vi "Main Listen for TCP Commands.vi"(8 "error in (no error)":errorcluster, 11 "J1939 Main Configuration":T1={"Parameters"={"J1939 XNET Settings"={"XNET Database"="", "XNET Cluster"="", "CAN Port"="", "Baud rate [Bd]"=0, "Termination"=0, "Incoming Rate"=0, "Outcoming Rate"=1, "Write Decimation"=1}, "Incoming Single Point Configuraiton"={"Incoming Single Point Frame"={"ID"=[], "Conversion"=[], "Channel Array Positions"=[], "Frame Length"=[]}, "Channel Pairs"={"Chan Refs"=[], "Previous Chan Values"=[]}, "Read FIFO"=refnum}, "Outgoing Cyclic Configuraiton"={"Outgoing Cyclic Frame"={"ID"=[], "Conversion"=[], "Channel Array Positions"=[], "Frame Length"=[], "Transmit Propreties"=[]}, "Channel Pairs"={"Block Data Refs"=[], "Previous Chan Values"=[]}, "Write FIFO"=refnum}, "J1939 Monitor Settings"={"J1939 Network Address"=0, "Name"=0}, "Simulated Addresses"=[], "Simulated Addresses LUT"=variant, "Name"=""}, "Name"="", "J1939 Cluster"={"Processed Incoming"=refnum, "Current Device Address"=0, "Processed Outgoing"=refnum, "Process Outgoing"=refnum, "Name"=0}, "References"={"BAM Buffer"=refnum, "CM Buffer"=refnum, "CM Gen"=refnum, "BAM Gen"=refnum, "Address Claims"=refnum, "RQST"=refnum}, "Frame In"="", "Frame Out"="", "Incoming Timeout"=0, "Outgoing Timeout"=0, "Listener ID"=refnum, "Process"=refnum, "Data Ref"=refnum, "Scale Ref"=refnum, "Incoming Direct Access"={"Offset"=0, "Length"=0}, "Outgoing Direct Access"={"Offset"=0, "Length"=0}, "TCP Mngr Ref"=refnum, "Name and Address"="", "Simulated Addresses"=[], "Simulated Addresses LUT"=variant} {"Simulated Addresses"."Simulated Addresses"."J1939 XNET Settings"."Name" format="%.0x"; "Simulated Addresses"."Simulated Addresses"."DM1 Data"."Data Reference" format="%.0x"; "Simulated Addresses"."Simulated Addresses"."DM1 Enable?"."Data Reference" format="%.0x"; "Simulated Addresses"."Simulated Addresses"."DM2 Data"."Data Reference" format="%.0x"; "Simulated Addresses"."Simulated Addresses"."DM2 Enable?"."Data Reference" format="%.0x"; "Parameters"."Simulated Addresses"."Simulated Addresses"."J1939 XNET Settings"."Name" format="%.0x"; "Parameters"."J1939 Monitor Settings"."Name" format="%.0x"; "Parameters"."Outgoing Cyclic Configuraiton"."Channel Pairs"."Block Data Refs"."Data Reference" format="%.0x"; "Parameters"."Outgoing Cyclic Configuraiton"."Outgoing Cyclic Frame"."Transmit Propreties"."Transmit Time" format="%#_p"; "Parameters"."J1939 XNET Settings"."Termination" items=["Off", "On"]; "Parameters"."Incoming Single Point Configuraiton"."Channel Pairs"."Chan Refs" format="%.0x"}) -> (0 "error out":errorcluster)   [LabVIEW 2015, in "J1939 Addon Engine.lvlib"]
uses:
  J1939 Addon Engine.lvlib
  Types/Configuration Cluster.ctl
  <vilib>/NI/NI VeriStand Inline Async API/_VS Inline Async API/Process/Process.lvclass
  Types/Process Parameters.ctl
  Shared/Types/XNET Settings.ctl
  Types/Incoming Single Point Configuration.ctl
  Types/Incoming Single Point Frame Pairs.ctl
  Shared/Types/Incoming Single Point Channel Pairs.ctl
  <vilib>/NI Veristand/Custom Device API/Data Reference.ctl
  Types/Outgoing Cyclic Configuration.ctl
  Types/Outgoing Cyclic Frame Pairs.ctl
  Shared/Types/XNET Frame Event Properties.ctl
  Shared/Types/Outgoing Cyclic Channel Pairs.ctl
  <vilib>/NI Veristand/Custom Device API/Block Data Reference.ctl
  Shared/Types/Monitor Settings.ctl
  Types/Simulated Settings.ctl
  Shared/Types/Compiled Simulated Settings.ctl
  Types/DTC FIFOs.ctl
  J1939 Multi Packet Frame/Types/Setup Information Cluster.ctl
  <vilib>/xnet/xnet.llb/XNET Frame CAN.ctl
  <vilib>/xnet/xnet.llb/XNET Frame Type CAN.ctl
  Shared/J1939 Utilities/Types/CAN Outgoing Message Cluster.ctl
  J1939 Multi Packet Frame/Types/TP List References.ctl
  J1939 Multi Packet Frame/Types/BAM Buffer Connections List_Ref.ctl
  J1939 Multi Packet Frame/Types/TP Buffer Connection Cluster.ctl
  J1939 Multi Packet Frame/Types/Connection Mode Generation Connection Ref.ctl
  J1939 Multi Packet Frame/Types/Connection Mode Generation Connection Cluster.ctl
  J1939 Multi Packet Frame/Types/BAM Generation Connections List_Ref.ctl
  J1939 Multi Packet Frame/Types/BAM Generation Connection Cluster.ctl
  J1939 Multi Packet Frame/Types/Address Table Reference.ctl
  J1939 Multi Packet Frame/Types/RQST Lookup Table Reference.ctl
  Types/Data Lookup Table Reference.ctl
  Types/Datatable Lookup DVR.ctl
  Types/Conversion Lookup Table Reference.ctl
  Shared/Types/RQST Comm Lookup Table_Ref.ctl
  Shared/STM/Connection Manager/stm_ManagerStateVariables.ctl
  Shared/STM/TCP/stm_TCP Connection Info.ctl
  Shared/STM/_SubVIs/stm_MetaDataElement.ctl
  Shared/STM/Connection Manager/stm_TCPConnectionProperties.ctl
  Shared/STM/Connection Manager/stm_TCPConnectionMethod.ctl
  Shared/STM/TCP/stm_TCP Read Options.ctl
  Shared/Types/Request Message.ctl
  J1939 Multi Packet Frame/Types/Address Lookup Table Action.ctl
  <vilib>/NI/NI VeriStand Inline Async API/_VS Inline Async API/Process/Process.lvclass/Process.ctl
  Shared/STM/TCP/STM Get Connection Reference (TCP).vi
  Shared/J1939 Utilities/Common Messages.vi
  Shared/J1939 Utilities/SubVIs/Request.vi
  J1939 Multi Packet Frame/SubVIs/RQST Lookup Table Act.vi
  <vilib>/NI/NI VeriStand Inline Async API/_VS Inline Async API/Error Handling Process/SubVIs/Error.ConvertArray.vi
  Shared/J1939 Utilities/Common Conversions.vi
  Shared/J1939 Utilities/SubVIs/Convert J1939 ID to CAN Arb ID.vi
  Shared/STM/Connection Manager/TCP Connection Manager.vi
  Shared/STM/TCP/STM Write Message (TCP).vi
  J1939 Multi Packet Frame/SubVIs/Address Lookup Table.vi
  <vilib>/xnet/xnet.llb/XNET Read (State CAN Comm).vi
  J1939 Multi Packet Frame/SubVIs/RQST Lookup Table.vi
  Shared/STM/TCP/STM Read Message (TCP).vi
  Shared/J1939 Addon Shared.lvlib
  Shared/J1939 Utilities/J1939 Utilities.lvlib
  <vilib>/NI Veristand/Custom Device Tools/Custom Device Utility Library/Custom Device Utility Library.lvlib
  <vilib>/NI VeriStand/Custom Device API/Custom Device API.lvlib
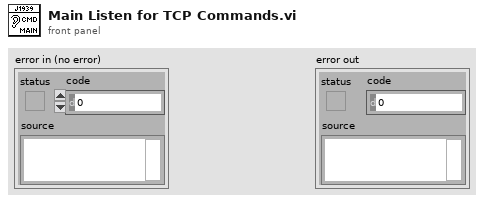
[diagram p1: front panel]
types:
  T1 = typedef "J1939 Addon Engine.lvlib/Configuration Cluster.ctl" = cluster{"Parameters":T2, "Name":string, "J1939 Cluster":T17, "References":T18, "Frame In":refnum<k21>, "Frame Out":refnum<k21>, "Incoming Timeout":u32, "Outgoing Timeout":u32, "Listener ID":refnum<k5>, "Process":refnum<class "Process.lvclass">, "Data Ref":T24, "Scale Ref":T25, "Incoming Direct Access":cluster{"Offset":u32, "Length":u32}, "Outgoing Direct Access":cluster{"Offset":u32, "Length":u32}, "TCP Mngr Ref":T26, "Name and Address":string, "Simulated Addresses":T14[], "Simulated Addresses LUT":variant}
  T2 = typedef "J1939 Addon Engine.lvlib/Process Parameters.ctl" = cluster{"J1939 XNET Settings":T3, "Incoming Single Point Configuraiton":T4, "Outgoing Cyclic Configuraiton":T8, "J1939 Monitor Settings":T13, "Simulated Addresses":T14[], "Simulated Addresses LUT":variant, "Name":string}
  T3 = typedef "J1939 Addon Shared.lvlib/XNET Settings.ctl" = cluster{"XNET Database":refnum<k21>, "XNET Cluster":refnum<k21>, "CAN Port":string, "Baud rate [Bd]":u32, "Termination":u32, "Incoming Rate":u32, "Outcoming Rate":u32, "Write Decimation":u32}
  T4 = typedef "J1939 Addon Engine.lvlib/Incoming Single Point Configuration.ctl" = cluster{"Incoming Single Point Frame":T5, "Channel Pairs":T6, "Read FIFO":refnum<k33>}
  T5 = typedef "J1939 Addon Engine.lvlib/Incoming Single Point Frame Pairs.ctl" = cluster{"ID":u32[], "Conversion":refnum<k21>[], "Channel Array Positions":cluster{"Offset":u32, "Length":u32}[], "Frame Length":u32[]}
  T6 = typedef "J1939 Addon Shared.lvlib/Incoming Single Point Channel Pairs.ctl" = cluster{"Chan Refs":T7[], "Previous Chan Values":dbl[]}
  T7 = typedef "Custom Device API.lvlib/Data Reference.ctl" = i32
  T8 = typedef "J1939 Addon Engine.lvlib/Outgoing Cyclic Configuration.ctl" = cluster{"Outgoing Cyclic Frame":T9, "Channel Pairs":T11, "Write FIFO":refnum<k33>}
  T9 = typedef "J1939 Addon Engine.lvlib/Outgoing Cyclic Frame Pairs.ctl" = cluster{"ID":u32[], "Conversion":refnum<k21>[], "Channel Array Positions":cluster{"Offset":u32, "Length":u32}[], "Frame Length":u32[], "Transmit Propreties":T10[]}
  T10 = typedef "J1939 Addon Shared.lvlib/XNET Frame Event Properties.ctl" = cluster{"Transmit trigger":enum16{"Channel value change"}, "Enable software cyclic trigger":bool, "Transmit Time":dbl}
  T11 = typedef "J1939 Addon Shared.lvlib/Outgoing Cyclic Channel Pairs.ctl" = cluster{"Block Data Refs":T12[], "Previous Chan Values":dbl[]}
  T12 = typedef "Custom Device API.lvlib/Block Data Reference.ctl" = cluster{"Data Reference":T7, "Offset":u64, "Length":u64}
  T13 = typedef "J1939 Addon Shared.lvlib/Monitor Settings.ctl" = cluster{"J1939 Network Address":u8, "Name":u64}
  T14 = typedef "J1939 Addon Engine.lvlib/Simulated Settings.ctl" = cluster{"Simulated Addresses":T15, "FIFOs":T16}
  T15 = typedef "J1939 Addon Shared.lvlib/Compiled Simulated Settings.ctl" = cluster{"J1939 XNET Settings":T13, "DM1 Data":T12[], "DM1 Data":dbl[], "DM1 Enable?":T12[], "DM1 Enable?":dbl[], "DM2 Data":T12[], "DM2 Data":dbl[], "DM2 Enable?":T12[], "DM2 Enable?":dbl[]}
  T16 = typedef "J1939 Addon Engine.lvlib/DTC FIFOs.ctl" = cluster{"DM1 Data":refnum<k33>, "DM1 Enable?":refnum<k33>, "DM2 Data":refnum<k33>, "DM2 Enable?":refnum<k33>, "DM1 Reset?":refnum<k33>, "DM2 Reset?":refnum<k33>}
  T17 = typedef "J1939 Addon Engine.lvlib/Setup Information Cluster.ctl" = cluster{"Processed Incoming":refnum<queue>, "Current Device Address":u8, "Processed Outgoing":refnum<queue>, "Process Outgoing":refnum<queue>, "Name":u64}
  T18 = typedef "J1939 Addon Engine.lvlib/TP List References.ctl" = cluster{"BAM Buffer":T19, "CM Buffer":T19, "CM Gen":T20, "BAM Gen":T21, "Address Claims":T22, "RQST":T23}
  T19 = typedef "J1939 Addon Engine.lvlib/BAM Buffer Connections List_Ref.ctl" = refnum<data-value>
  T20 = typedef "J1939 Addon Engine.lvlib/Connection Mode Generation Connection Ref.ctl" = refnum<data-value>
  T21 = typedef "J1939 Addon Engine.lvlib/BAM Generation Connections List_Ref.ctl" = refnum<data-value>
  T22 = typedef "J1939 Addon Engine.lvlib/Address Table Reference.ctl" = refnum<data-value>
  T23 = typedef "J1939 Addon Engine.lvlib/RQST Lookup Table Reference.ctl" = refnum<data-value>
  T24 = typedef "J1939 Addon Engine.lvlib/Data Lookup Table Reference.ctl" = refnum<data-value>
  T25 = typedef "J1939 Addon Engine.lvlib/Conversion Lookup Table Reference.ctl" = refnum<data-value>
  T26 = typedef "J1939 Addon Shared.lvlib/RQST Comm Lookup Table_Ref.ctl" = refnum<data-value>
  T27 = typedef "J1939 Addon Shared.lvlib/stm_TCPConnectionMethod.ctl" = enum16{"Initialize", "Add Connection", "Set Properties", "Get Connection(s)", "Remove Connection", "Remove All Connections", "Get Connection Count"}
  T28 = typedef "J1939 Addon Shared.lvlib/stm_TCP Read Options.ctl" = cluster{"Ignore Timeout Error":bool, "timeout ms (1000)":i32}
  T29 = typedef "J1939 Addon Shared.lvlib/Request Message.ctl" = cluster{"PGN":u32, "DA":u8, "Ignore Response":bool}
  T30 = typedef "J1939 Addon Shared.lvlib/J1939 Utilities.lvlib/CAN Outgoing Message Cluster.ctl" = cluster{"Identifier":u32, "Data":u8[]}
  T31 = typedef "J1939 Addon Engine.lvlib/Address Lookup Table Action.ctl" = enum16{"Initialize", "Add", "Get", "Remove", "Get All"}
  T32 = typedef "J1939 Addon Shared.lvlib/stm_TCP Connection Info.ctl" = cluster{"connection ID":refnum<k5>, "Meta data":T33[]}
  T33 = typedef "J1939 Addon Shared.lvlib/stm_MetaDataElement.ctl" = string
  T34 = typedef "XNET Frame CAN.ctl" = cluster{"timestamp":timestamp, "payload":u8[], "identifier":u32, "type":T35, "extended?":bool, "echo?":bool}
  T35 = typedef "XNET Frame Type CAN.ctl" = u8
  T36 = typedef "XNET CAN Comm.ctl" = cluster{"fault code":i32, "fault?":bool, "communication state":T37, "last error":T38, "receive error counter":u8, "transmit error counter":u8, "transceiver error?":bool, "sleep?":bool}
  T37 = typedef "XNET CAN Comm State.ctl" = u8
  T38 = typedef "XNET CAN Last Err.ctl" = u8
  T39 = typedef "J1939 Addon Shared.lvlib/Address Lookup Table Data.ctl" = cluster{"Name":u8[], "Address":u8}
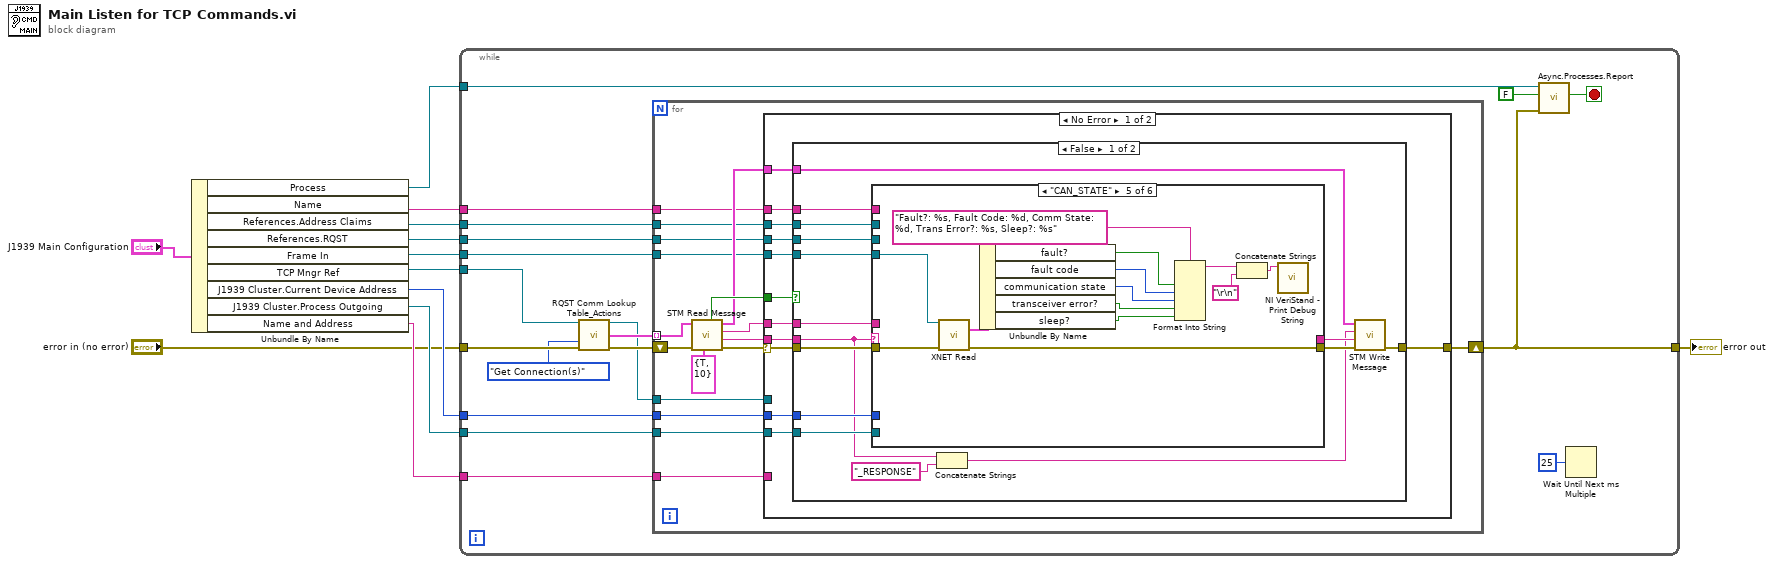
[diagram p0: block diagram]
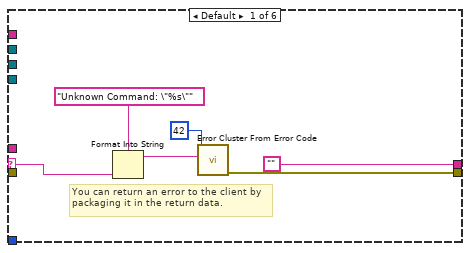
[diagram p2: hidden frame]
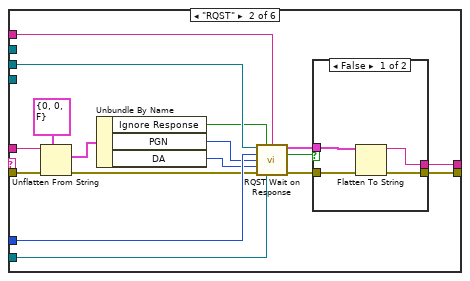
[diagram p3: hidden frame]
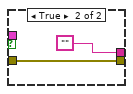
[diagram p4: hidden frame]
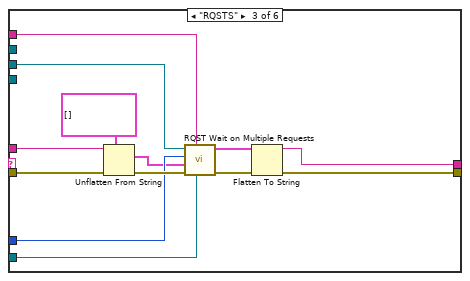
[diagram p5: hidden frame]
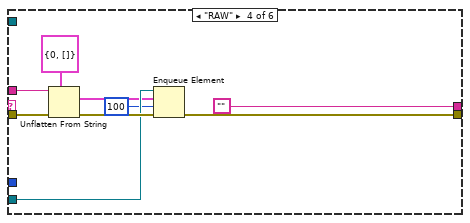
[diagram p6: hidden frame]
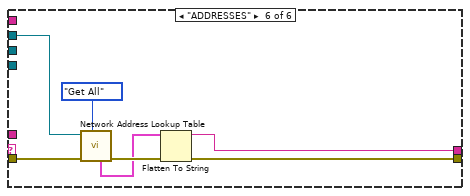
[diagram p7: hidden frame]
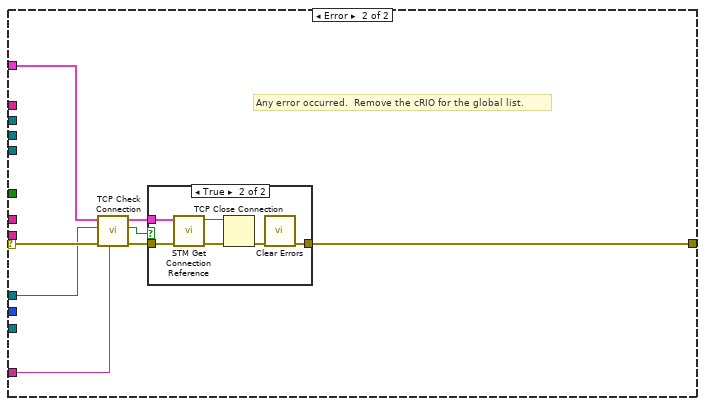
[diagram p9: hidden frame]
diagram:
  n1 = Unbundle By Name("J1939 Main Configuration") -> ("Process"=w12:refnum<class "Process.lvclass">, "Name"=w11:string, "References.Address Claims"=w10:T22, "References.RQST"=w9:T23, "Frame In"=w8:refnum<k21>, "TCP Mngr Ref"=w7:T26, "J1939 Cluster.Current Device Address"=w6:u8, "J1939 Cluster.Process Outgoing"=w5:refnum<queue>, "Name and Address"=w4:string)
  n2 = while {
    tunnel: "error in (no error)" -> [w27]
    tunnel: [w13] -> w1
    tunnel: w12 -> [w29]
    tunnel: w7 -> [w26]
    tunnel: w11 -> [w25]
    tunnel: w4 -> [w24]
    tunnel: w8 -> [w23]
    tunnel: w5 -> [w17]
    tunnel: w6 -> [w16]
    tunnel: w9 -> [w15]
    tunnel: w10 -> [w14]
    stop <- w30 stop-if-true
    n3 = call "RQST Comm Lookup Table_Actions.vi"("ref in"=w26, "Method"=stm_TCPConnectionMethod."Get Connection(s)", "error in (no error)"=w27) -> ("reference out"=w18:T26, "All Connections"=w19:T32[], "error out"=w21:errorcluster)  [unwired: 6 in, 4 out]
    n4 = for {
      tunnel: w19 -> [w47] mode=indexing
      shift-right: [w43] -> w13
      shift-left: w21 -> [w42]
      tunnel: w15 -> [w38]
      tunnel: w14 -> [w37]
      tunnel: w17 -> [w36]
      tunnel: w16 -> [w35]
      tunnel: w18 -> [w34]
      tunnel: w25 -> [w33]
      tunnel: w24 -> [w32]
      tunnel: w23 -> [w31]
      n5 = call-poly "STM Read Message.vi"("Options"=T28 {"Ignore Timeout Error"=TRUE, "timeout ms (1000)"=10}, "error in"=w42, "Connection In"=w47) -> ("error out"=w41:errorcluster, "Name"=w44:T33, "data string"=w45:string, "Connection In"=w40:T32, "Timed Out?"=w46:bool)  [unwired: 3 in, 1 out]
      n6 = case shown="No Error" w41 {
        selector: w41 -> [w55 w154]
        tunnel: w46 -> [w59 _]
        tunnel: w45 -> [w58 _]
        tunnel: w44 -> [w57 _]
        tunnel: [w56 w149] -> w43
        tunnel: w40 -> [w50 w153]
        tunnel: w38 -> [w54 _]
        tunnel: w37 -> [w53 _]
        tunnel: w36 -> [w52 _]
        tunnel: w35 -> [w51 _]
        tunnel: w34 -> [_ w148]
        tunnel: w33 -> [w49 _]
        tunnel: w32 -> [_ w147]
        tunnel: w31 -> [w48 _]
        frame No Error {
          n7 = case shown="False" w59 {
            tunnel: w58 -> [w73 _]
            tunnel: w57 -> [w63 _]
            tunnel: w55 -> [w74 w146]
            tunnel: [w66 w146] -> w56
            tunnel: w54 -> [w72 _]
            tunnel: w53 -> [w71 _]
            tunnel: w52 -> [w70 _]
            tunnel: w51 -> [w69 _]
            tunnel: w50 -> [w65 _]
            tunnel: w49 -> [w61 _]
            tunnel: w48 -> [w60 _]
            frame False {
              n8 = case shown="\"CAN_STATE\"" w63 {
                selector: w63 -> [w76 _ _ _ _ _]
                tunnel: w73 -> [_ w84 w113 w124 _ _]
                tunnel: [w77 w96 w116 w118 w136 w139] -> w67
                tunnel: ["" ("data string") w93 w115 "" _ w140] -> w68
                tunnel: w70 -> [_ w91 w110 w121 _ _]
                tunnel: w74 -> [_ w90 w114 w125 w138 w144]
                tunnel: w72 -> [_ w83 w108 _ _ _]
                tunnel: w69 -> [_ w97 w107 _ _ _]
                tunnel: w71 -> [_ _ _ _ _ w143]
                tunnel: w61 -> [_ w81 w104 _ _ _]
                tunnel: w60 -> [_ _ _ _ w137 _]
                frame Default {
                  # "You can return an error to the client by packaging it in the return data."
                  n9 = Format Into String(format string="Unknown Command: \"%s\"", w76) -> (resulting string=w78:string)  [unwired: 2 in, 1 out]
                  n10 = call <vilib>:"Error Cluster From Error Code.vi"("error message (\"\")"=w78, "error code (0)"=42) -> ("error out"=w77:errorcluster)  [unwired: 7 in]
                }
                frame "RQST" {
                  n11 = Unflatten From String(type=T29 {"PGN"=0, "DA"=0, "Ignore Response"=FALSE} ("Cluster"), binary string=w84, error in (no error)=w90) -> (value=w87:T29, error out=w89:errorcluster)  [unwired: 2 in, 1 out]
                  n12 = Unbundle By Name(w87) -> ("Ignore Response"=w82:bool, "PGN"=w86:u32, "DA"=w85:u8)
                  n13 = call "RQST Wait on Response.vi"("ref in"=w83, "Ignore Response"=w82, "Name"=w81, "Source Address"=w97, "PGN"=w86, "DA"=w85, "error in (no error)"=w89, "Processed Outgoing"=w91) -> ("element"=w92:T34, "timed out?"=w94:bool, "error out"=w95:errorcluster)  [unwired: 4 in, 1 out]
                  n14 = case shown="False" w94 {
                    tunnel: [w99 w103] -> w96
                    tunnel: w95 -> [w100 w103]
                    tunnel: [w98 ""] -> w93
                    tunnel: w92 -> [w101 _]
                    frame False {
                      n15 = Flatten To String(anything=w101, error in (no error)=w100) -> (data string=w98:string, error out=w99:errorcluster)  [unwired: 2 in, 1 out]
                    }
                    frame True {
                    }
                  }
                }
                frame "RQSTS" {
                  n16 = Unflatten From String(type=T29[] [], binary string=w113, error in (no error)=w114) -> (value=w106:T29[], error out=w111:errorcluster)  [unwired: 2 in, 1 out]
                  n17 = call "RQST Wait on Multiple Requests.vi"("Processed Outgoing"=w110, "Name"=w104, "error in (no error)"=w111, "value"=w106, "Source Address"=w107, "ref in"=w108) -> ("error out"=w109:errorcluster, "Elements"=w105:T34[])  [unwired: 2 in, 2 out]
                  n18 = Flatten To String(anything=w105, error in (no error)=w109) -> (data string=w115:string, error out=w116:errorcluster)  [unwired: 2 in, 1 out]
                }
                frame "RAW" {
                  n19 = Unflatten From String(type=T30 {"Identifier"=0, "Data"=[]} ("Data to Send"), binary string=w124, error in (no error)=w125) -> (value=w120:T30, error out=w122:errorcluster)  [unwired: 2 in, 1 out]
                  n20 = Enqueue Element(queue=w121, element=w120, timeout in ms (-1)=100, error in (no error)=w122) -> (error out=w118:errorcluster)  [unwired: 2 out]
                }
                frame "CAN_STATE" {
                  n21 = call-poly <vilib>:"XNET Read.vi"("session in"=w137, "error in (no error)"=w138) -> ("CAN comm"=w135:T36, "error out"=w136:errorcluster)  [unwired: 11 in, 1 out]
                  n22 = Unbundle By Name(w135) -> ("fault?"=w134:bool, "fault code"=w133:i32, "communication state"=w132:T37, "transceiver error?"=w131:bool, "sleep?"=w130:bool)
                  n23 = Format Into String(format string="Fault?: %s, Fault Code: %d, Comm State: %d, Trans Error?: %s, Sleep?: %s", w134, w133, w132, w131, w130) -> (resulting string=w129:string)  [unwired: 2 in, 1 out]
                  n24 = Concatenate Strings(w129, "\r\n") -> (w127:string)
                  n25 = call <vilib>:"NI VeriStand - Print Debug String.vi"("Message"=w127) -> ()  [unwired: 10 in, 1 out]
                }
                frame "ADDRESSES" {
                  n26 = call "Network Address Lookup Table.vi"("Action"=Address_Lookup_Table_Action."Get All", "error in (no error)"=w144, "Address LUT"=w143) -> ("error out"=w142:errorcluster, "All Data"=w141:T39[])  [unwired: 4 in, 3 out]
                  n27 = Flatten To String(anything=w141, error in (no error)=w142) -> (data string=w140:string, error out=w139:errorcluster)  [unwired: 2 in, 1 out]
                }
              }
              n28 = Concatenate Strings(w63, "_RESPONSE" ("string")) -> (w62:string)
              n29 = call-poly "STM Write Message.vi"("error in (no error)"=w67, "Data"=w68, "Name"=w62, "Connection Info"=w65) -> ("error out"=w66:errorcluster)  [unwired: 6 in, 1 out]
            }
            frame True {
              # "No Message."
            }
          }
        }
        frame Error {
          # "Any error occurred.  Remove the cRIO for the global list."
          n30 = call "TCP Check Connection.vi"("Name"=w147, "error in (no error)"=w154, "ref in"=w148, "Connection In"=w153) -> ("error out"=w150:errorcluster, "Disconnected"=w152:bool, "Connection out"=w151:T32)  [unwired: 5 in]
          n31 = case shown="True" w152 {
            tunnel: [w155 w158] -> w149
            tunnel: w150 -> [w155 w161]
            tunnel: w151 -> [_ w156]
            frame False {
            }
            frame True {
              n32 = call-poly "STM Get Connection Reference.vi"("error in"=w161, "Connection Info"=w156) -> ("error out"=w160:errorcluster, "connection ID out"=w159:refnum<k5>)  [unwired: 7 in, 1 out]
              n33 = TCP Close Connection(connection ID=w159, error in (no error)=w160) -> (error out=w157:errorcluster)  [unwired: 1 in, 1 out]
              n34 = call <vilib>:"Clear Errors.vi"("error in (no error)"=w157) -> ("error out"=w158:errorcluster)  [unwired: 5 in, 1 out]
            }
          }
        }
      }
    }
    n35 = call <vilib>:"Async.Processes.Report.vi"("Error"=w13, "Stop on Error?"=FALSE, "Process in"=w29) -> ("Stop"=w30:bool)  [unwired: 7 in, 1 out]
    n36 = Wait Until Next ms Multiple(millisecond multiple=u32 25) -> ()  [unwired: 1 out]
  }
  "error out" <- w1
